vi "Construct Sequence.vi"(8 "error in":errorcluster, 11 "Sequence Builder in":refnum<class "Sequence Builder.lvclass">) -> (0 "error out":errorcluster, 2 "New Sequence":refnum<class "SEQ.lvclass">, 3 "Sequence Builder out":refnum<class "Sequence Builder.lvclass">)   [LabVIEW 2014, in "Sequence Builder.lvclass"]
doc: "Construct a new sequence using the builder class."
uses:
  Sequence Builder.lvclass
  SEQ/SEQ.lvclass
  SEQ/SEQ.lvclass/SEQ.ctl
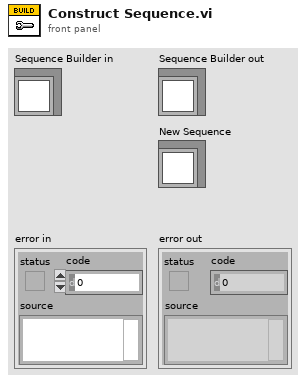
[diagram p1: front panel]
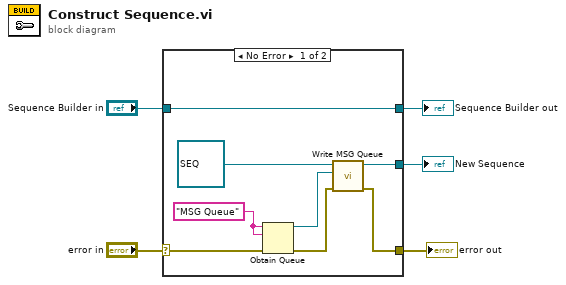
[diagram p0: block diagram]
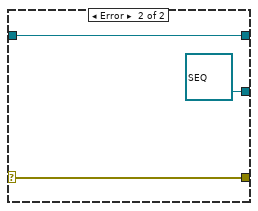
[diagram p2: hidden frame]
diagram:
  n1 = case shown="No Error" "error in" {
    selector: "error in" -> [w11 w16]
    tunnel: [w6 w16] -> w4
    tunnel: [w13 w15] -> w2
    tunnel: "Sequence Builder in" -> [w13 w15]
    tunnel: [w8 refnum<class "SEQ.lvclass"> refnum ("SEQ out")] -> w1
    frame No Error {
      w12 = "MSG Queue" ("name (unnamed)")
      n2 = Obtain Queue(name (unnamed)=w12, element data type=w12, error in (no error)=w11) -> (queue out=w9:refnum<queue>, error out=w7:errorcluster)  [unwired: 2 in, 1 out]
      n3 = call "Write MSG Queue.vi"("error in (no error)"=w7, "MSG Queue"=w9, "SEQ in"=refnum<class "SEQ.lvclass"> refnum ("Sequence Composition:SEQ")) -> ("error out"=w6:errorcluster, "SEQ out"=w8:refnum<class "SEQ.lvclass">)  [unwired: 7 in]
    }
    frame Error {
    }
  }
  "error out" <- w4
  "Sequence Builder out" <- w2
  "New Sequence" <- w1
